vi "Configure Channel (AIDI Delta).vi"(0 "VISA resource name":refnum<visa-resource-name>, 1 "Reference Channel (1)":string="0001", 5 "Channel (0001)":string="0001", 7 "Enable Channel (True)":bool=TRUE, 9 "Span":T1={"DI Type (0 : LVL)"=0, "Lower Span (0)"=0, "Upper Span (1)"=1} {"Upper Span (1)" min=-99999 max=99999 step=1; "Lower Span (0)" min=-99999 max=99999 step=1; "DI Type (0 : LVL)" items=["LVL", "DI"]}, 11 "error in (no error)":errorcluster) -> (4 "VISA resource name out":refnum<visa-resource-name>, 6 "Channel":string, 15 "error out":errorcluster)   [LabVIEW 2020, in "Yokogawa GX Series.lvlib"]
doc: "Sets the input range as Contact.\n\nCommand: SRangeAI"
uses:
  <instrlib>/Yokogawa GX Series/Yokogawa GX Series.lvlib
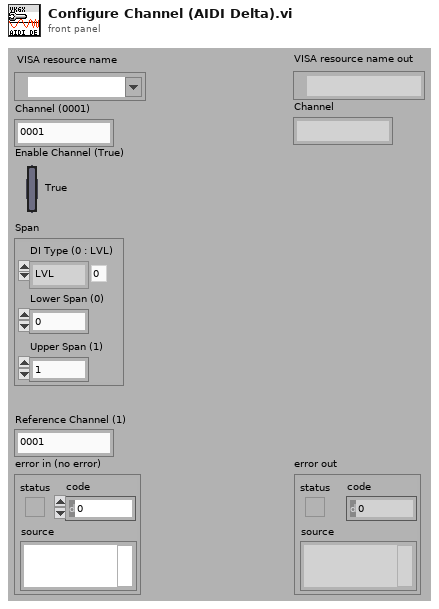
[diagram p1: front panel]
types:
  T1 = cluster{"DI Type (0 : LVL)":i32, "Lower Span (0)":i32, "Upper Span (1)":i32}
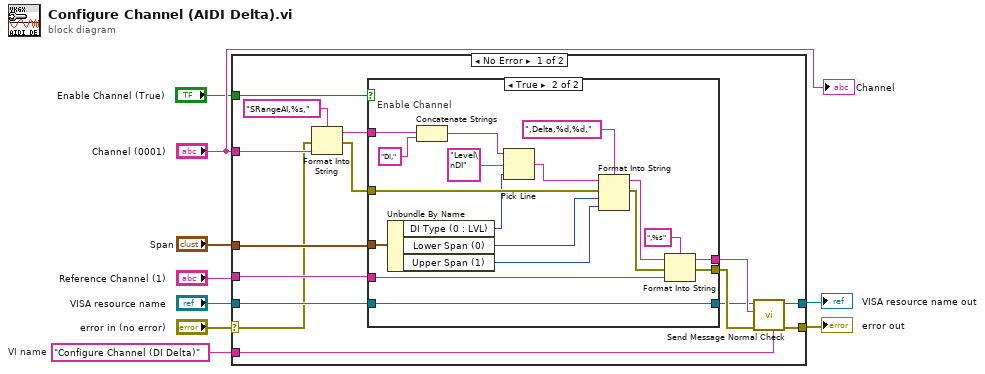
[diagram p0: block diagram]
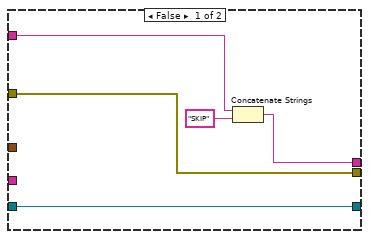
[diagram p2: hidden frame]
diagram:
  w8 = "Configure Channel (DI Delta)"  # VI name
  n1 = case shown="No Error" "error in (no error)" {
    selector: "error in (no error)" -> [w10 w48]
    tunnel: "Reference Channel (1)" -> [w21 _]
    tunnel: w8 -> [w18 _]
    tunnel: [w17 w49] -> w7
    tunnel: [w16 w48] -> w6
    tunnel: "Span" -> [w15 _]
    tunnel: "Channel (0001)" -> [w14 _]
    tunnel: "VISA resource name" -> [w13 w49]
    tunnel: "Enable Channel (True)" -> [w11 _]
    frame No Error {
      n2 = Format Into String(format string="SRangeAI,%s,", error in=w10, w14) -> (resulting string=w22:string, error out=w23:errorcluster)  [unwired: 1 in]
      n3 = case shown="True" w11 {
        tunnel: w23 -> [w26 w46]
        tunnel: w22 -> [w27 w44]
        tunnel: w21 -> [_ w42]
        tunnel: [w26 w38] -> w20
        tunnel: [w28 w37] -> w19
        tunnel: w15 -> [_ w34]
        tunnel: [w25 w30] -> w12
        tunnel: w13 -> [w25 w30]
        frame False {
          n4 = Concatenate Strings(w27, "SKIP") -> (w28:string)
        }
        frame True {
          # "Enable Channel"
          n5 = Unbundle By Name(w34) -> ("DI Type (0 : LVL)"=w33:i32, "Lower Span (0)"=w32:i32, "Upper Span (1)"=w31:i32)
          n6 = Concatenate Strings(w44, "DI,") -> (w36:string)
          n7 = Pick Line(string ("")=w36, multi-line string="Level\nDI", line index=w33) -> (output string=w43:string)
          n8 = Format Into String(format string=",Delta,%d,%d,", initial string=w43, error in=w46, w32, w31) -> (resulting string=w39:string, error out=w40:errorcluster)
          n9 = Format Into String(format string=",%s", initial string=w39, error in=w40, w42) -> (resulting string=w37:string, error out=w38:errorcluster)
        }
      }
      n10 = call <instrlib>:"Send Message Normal Check.vi"("Source (\"\")"=w18, "error in (no error)"=w20, "Send Message (\"\")"=w19, "VISA resource name"=w12) -> ("error out"=w16:errorcluster, "VISA resource name out"=w17:refnum<visa-resource-name>)  [unwired: 2 in, 4 out]
    }
    frame Error {
    }
  }
  "error out" <- w6
  "VISA resource name out" <- w7
  "Channel" <- "Channel (0001)"
